vi "Extract Image Rect.vi"(6 "Zone H":dbl=7.0 format="%#_13g", 8 "Zone W":dbl=7.0 format="%#_13g", 9 "Exam Zone Offset Y":dbl, 10 "Exam Zone Offset X":dbl, 11 "Source In":T1) -> (2 "Extracted Out":T1, 3 "Annotated Source Out":T1)   [LabVIEW 2014]
uses:
  <vilib>/vision/Image Controls.llb/IMAQ Image.ctl
  <vilib>/vision/NI_Vision_Development_Module.lvlib
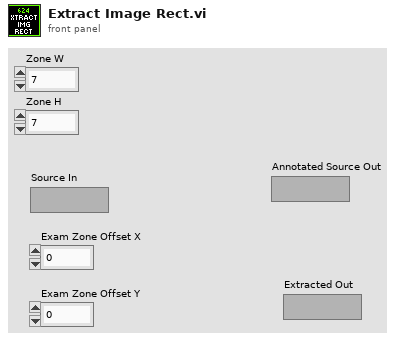
[diagram p1: front panel]
types:
  T1 = typedef "IMAQ Image.ctl" = refnum<image>
  T2 = cluster{"[0]":i32, "[1]":i32, "[2]":i32, "[3]":i32}
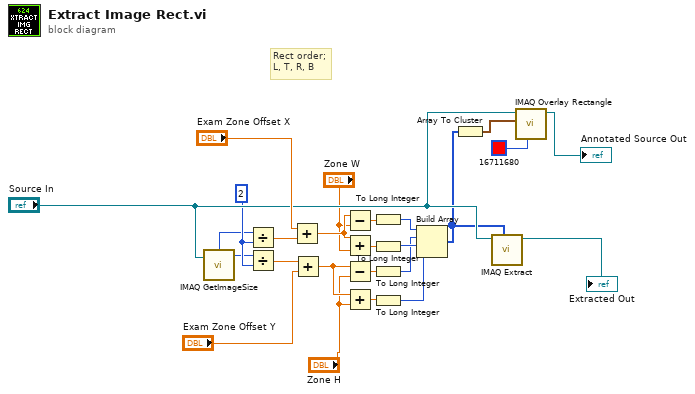
[diagram p0: block diagram]
diagram:
  w4 = 2 ("y")
  # "Rect order;\nL, T, R, B"
  n1 = call "IMAQ GetImageSize"("Image"="Source In") -> ("Y Resolution"=w3:i32, "X Resolution"=w2:i32)  [unwired: 3 in, 1 out]
  n2 = Divide(x=w2, y=w4) -> (x/y=w19:dbl)
  n3 = Divide(x=w3, y=w4) -> (x/y=w21:dbl)
  n4 = Add(x="Exam Zone Offset X", y=w19) -> (x+y=w24:dbl)
  n5 = Add(x=w21, y="Exam Zone Offset Y") -> (x+y=w23:dbl)
  n6 = Subtract(x=w24, y="Zone W") -> (x-y=w6:dbl)
  n7 = Add(x=w24, y="Zone W") -> (x+y=w13:dbl)
  n8 = Subtract(x=w23, y="Zone H") -> (x-y=w7:dbl)
  n9 = Add(x=w23, y="Zone H") -> (x+y=w8:dbl)
  n10 = To Long Integer(number=w6) -> (32bit integer=w9:i32)
  n11 = To Long Integer(number=w13) -> (32bit integer=w11:i32)
  n12 = To Long Integer(number=w7) -> (32bit integer=w10:i32)
  n13 = To Long Integer(number=w8) -> (32bit integer=w12:i32)
  n14 = Build Array(w9, w10, w11, w12) -> (w14:i32[])
  n15 = Array To Cluster(array=w14) -> (cluster=w15:T2)
  n16 = call "IMAQ Extract"("Optional Rectangle"=w14, "Image Src"="Source In") -> ("Image Dst Out"=→"Extracted Out":T1)  [unwired: 8 in, 1 out]
  n17 = call "IMAQ Overlay Rectangle"("Color"=u32 16711680, "Rectangle"=w15, "Image"="Source In") -> ("Image Out"=→"Annotated Source Out":T1)  [unwired: 7 in, 1 out]
